vi "HEWH RLT PRAT.vi"() -> ()   [LabVIEW 2023] (continued)
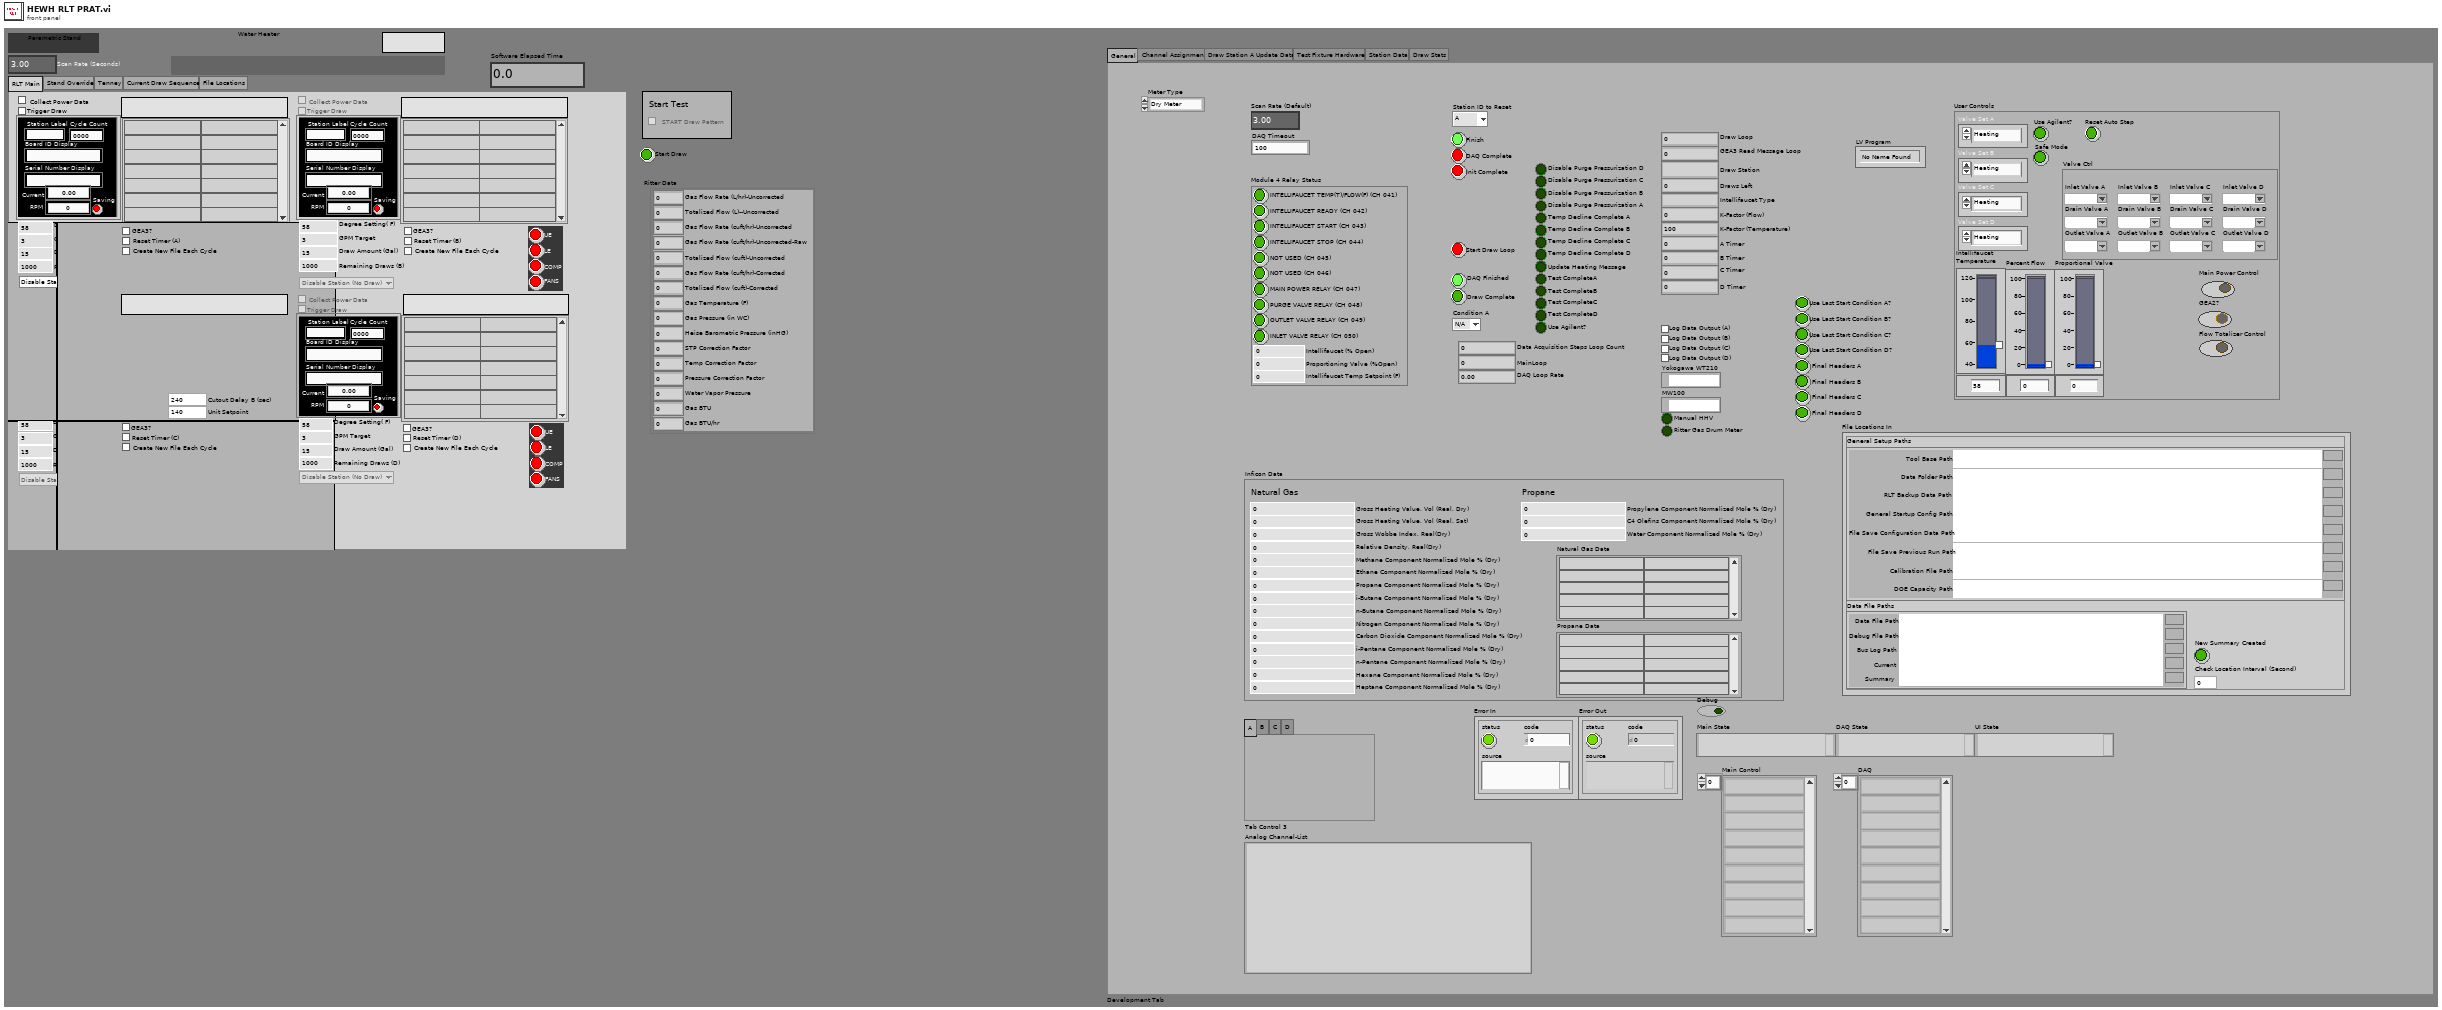
[diagram p1: front panel]
types:
  T1 = typedef "Ritter Data.ctl" = cluster{"Gas Flow Rate (L/hr)-Uncorrected":dbl, "Totalized Flow (L)--Uncorrected":dbl, "Gas Flow Rate (cuft/hr)-Uncorrected":dbl, "Totalized Flow (cuft)-Uncorrected":dbl, "Gas Temperature (F)":dbl, "Gas Pressure (in WC)":dbl, "Heise Barometric Pressure (inHG)":dbl, "STP Correction Factor":dbl, "Temp Correction Factor":dbl, "Pressure Correction Factor":dbl, "Water Vapor Pressure":dbl, "Gas Flow Rate (cuft/hr)-Corrected":dbl, "Totalized Flow (cuft)-Corrected":dbl, "Gas BTU":dbl, "Gas BTU/hr":dbl, "Gas Flow Rate (cuft/hr)-Uncorrected-Raw":dbl}
  T2 = typedef "HEWH Special Condition Check.ctl" = enum16{"N/A", "C1", "C2", "Reset/Fail", "Skip Draw Sequence"}
  T3 = typedef "File Setup.lvlib/Save File DOE File Path Control.ctl" = cluster{"General Setup Paths":cluster{"Calibration File Path":path, "DOE Capacity Path":path, "Data Folder Path":path, "RLT Backup Data Path":path, "Tool Base Path":path, "General Startup Config Path":path, "File Save Previous Run Path":path, "File Save Configuration Data Path":path}, "Data File Paths":T4, "New Summary Created":bool, "Check Location Interval (Second)":i32}
  T4 = typedef "File Setup.lvlib/Save File DOE Data Save Filepaths.ctl" = cluster{"Data File Path":path, "Debug File Path":path, "Bus Log Path":path, "Current":path, "Summary":path}
  T5 = typedef "File Setup.lvlib/Save File DISH Dishwasher Details.ctl" = cluster{"FileVersionInfo":T6, "Dishwasher Info":cluster{"Open Cup Weight (gm):":dbl, "Auto Cup Weight (gm):":dbl, "Detergent-Dish:":string, "Inlet Temperature-Dish:":string, "Cycle Mode-Dish:":string, "Unit Control-Dish:":string, "Manufacturer-Dish:":string}, "Washer Info":cluster{"Hot Water Temperature (Fahrenheit):":string, "Cold Water Temperature (Fahrenheit):":string, "Capacity (cu.ft):":dbl, "Initial Cloth Weight:":dbl, "Cloth Lot:":i32, "Model Family:":string, "Program Name:":string, "Cycle Selection:":string, "Wash Temperature:":string, "Rinse Temperature:":string, "Load Size:":string}, "File Name Output Array":string[][], "Calibration Output Array":string[][], "Appliance Common":T7, "Water Heater":cluster{"Heating Mode:":string}, "Dryer":cluster{"Heat Setting:":T8, "Washer Water Temperature (60 ± 5°F):":u16, "Water Hardness (PPM):":u16, "Dryness Setting:":T8, "Dryer Type:":string, "Exhaust:":string, "Drying Cycle:":string, "Load Type:":string, "Nominal Load Weight":string, "Dryer Initial IMC Data":T9}}
  T6 = typedef "FileVersionInformation.ctl" = cluster{"FileVersion":string, "ProductName":string, "InternalName":string, "CompanyName":string, "LegalCopyright":string, "FileDescription":string}
  T7 = typedef "DOE Appliance Common.ctl" = cluster{"Engineer:":string, "Model Number:":string, "Serial Number:":string, "Comments:":string, "Station ID:":string, "Technician:":string, "TR Number:":string, "Lab ID:":string, "Voltage:":string, "Water Pressure (PSI):":string, "Test Date:":string, "Computer Name:":string, "IP Address:":string, "Ambient RH:":string, "Frequency:":string, "Build:":string, "Filename:":string, "Test Type:":string, "Load Run #:":i32, "Ambient Temperature (F):":string, "File Path:":path, "Cycles Per Year":u32}
  T8 = typedef "Custom Pallet String.ctl" = string
  T9 = typedef "DPT IMC Data.ctl" = cluster{"Measured IMC (lbs)":dbl, "Actual Initial RMC (%)":dbl, "RMC (Desired %)":dbl, "Bone Dry Wt(lbs)":dbl, "Tolerance(%)":dbl, "Actual Final RMC (%)":dbl, "CEF (lbf/kWh)":dbl, "Minimum Weight (lbf)":dbl, "Average Weight (lbf)":dbl, "Maximum Weight (lbf)":dbl, "Measured IMC In Range?":bool, "Moisture Reduction Factor":dbl, "Field Use Factor":dbl, "Empty Dryer Cold Weigth":dbl, "Energy Standard":T10, "Weight Cloth (lbs)":dbl, "Relative Moisture Content (%)":dbl, "Relative Moisture Content - Avg (%)":dbl}
  T10 = typedef "DOE Dryer Standard.ctl" = enum16{"D2-Automatic Dryer", "D2-Timer Dryer", "D1-Automatic Dryer", "D1-Timer Dryer", "Other"}
  T11 = typedef "Custom Pallet DBL.ctl" = dbl
  T12 = typedef "UTILITY Power Analyzer.ctl" = enum16{"", "APLUS", "WT210", "WT500", "WT300", "OSI", "Debug", "WT230", "WT300_1", "WT300_2"}
  T13 = typedef "HEWH Output Information.ctl" = cluster{"Scan Rate Adjust":dbl, "Draw Count":i32, "Test Patten Setup":T14, "HEWH Specific DAQ":T21, "Test Output Data":cluster{"PreDraw Data Table":string[][], "Data Table":string[][], "MW100 TC Headers":string[]}, "Calc and Calibration":T24, "Current Draw Time":dbl, "LV Program":T25, "Station ID":T26, "Current Cond":T2, "Test Complete":bool, "ANSI Rate":T27, "Module 4 Relay Status":T28}
  T14 = typedef "HEWH Draw Pattern Setup.ctl" = cluster{"Total Gallons Schedule":dbl[], "PRAT/RLT Sequence":T15[], "Current Sequence Index":i32}
  T15 = typedef "PRAT Test.ctl" = cluster{"Sequence #":dbl, "Cycles":i32, "Mode Setting":T16, "Flow Rate (GPM)":dbl, "Temperature (F)":dbl, "Reset Timer":bool, "Use Temp Decline Method":bool, "Terminate Condition":T17, "Condition Value #1":dbl, "UE":bool, "LE":bool, "Comp":bool, "Fan":bool, "Test End Time (Sec)":dbl, "Purge Until Cutout":bool, "Start Conditions":T18, "Condition Value #2":dbl, "Remove Power":bool, "Time":dbl, "Check Special Cond.":T19, "Condition#":T2, "Draw Flags":T20, "Data Processing Delay (FHD 15sec, UEF 5 Sec)":dbl, "Test Complete":bool, "User Setpoint":dbl, "Tank Setpoint":dbl}
  T16 = typedef "File Setup.lvlib/Save File HEWH Heating Control Mode.ctl" = string
  T17 = typedef "Terminate Draw Conditions.ctl" = enum16{"C1-Terminate Draw @ Gallon Mark", "C2-Special Last Draw (HU Test)", "C3-RTD Out <=", "C4-Mean Tank Temp <=", "C5-Decrease RTD Out (Deg F)", "C6-Time (Seconds)", "C7-Until Any Heat Source", "C8-Specific Heat Source", "C9-Do Nothing", "C10-Inlet Outlet RTD Temp Delta"}
  T18 = typedef "HEWH Start Conditions.ctl" = enum16{"Heat Source Cutout", "At Time (Seconds)", "Every X (Seconds)", "T2 >= X° Below Setpoint", "Seconds From Complete", "Wait for LE & Comp Cutout", "Wait for Comp Cutout", "Wait for LE Cutout", "Wait for UE Cutout", "Start Immediately"}
  T19 = typedef "Check Special Condtions.ctl" = enum16{"SC1-Do Nothing", "SC2-Check Heat Source (On-C2/Off-C1)", "SC3-Check Skip Condition", "SC4-Check Heat Source ON/Fail", "SC5-Keep Draw Valves Open", "SC6-Skip Purge"}
  T20 = typedef "HEWH Draw Flag ENUM.ctl" = enum16{"N/A", "None(0)", "Sml(1)", "Med(2)", "SmlMed(3)", "Lrg(4)", "SmlLrg(5)", "MedLrg(6)", "SmlMedLrg(7)"}
  T21 = typedef "HEWH Specific DAQ.ctl" = cluster{"HEWH Data":T22, "Flow Valve % Open":dbl, "Power State":T23, "Power Analyzer":T12, "Flow Valve uA Output":i32, "Gallons Start (Gal)":dbl, "PI Output":dbl}
  T22 = typedef "HEWH Power Data.ctl" = cluster{"HEWH Standard":cluster{"Voltage (Volts)":dbl, "Current (Amps)":dbl, "Power (Watts)":dbl, "WattHours (Wh)":dbl, "TC Tree (AVG)":dbl, "Flow Rate (GPM)":dbl, "Gallons (Gal)":dbl, "RTD Out (Deg F)":dbl, "RTD In (Deg F)":dbl, "RTD Amb (Deg F)":dbl, "TC Down":dbl, "UE Event Lead":i32, "LE Event Lead":i32, "TC 8":dbl, "TC 9":dbl, "TC 10":dbl, "TC Tree Array (1-6)":dbl[], "TC 7":dbl, "PSI 1":dbl, "PSI 2":dbl, "PSI 3":dbl, "PSI 4":dbl}, "PRAT":cluster{"Power (Watts) A":dbl, "Power (Watts) B":dbl, "Power (Watts) C":dbl, "Power (Watts) D":dbl, "TC1":dbl, "TC2":dbl, "TC3":dbl, "TC4":dbl, "WattHours (Wh) A":dbl, "WattHours (Wh) B":dbl, "WattHours (Wh) C":dbl, "WattHours (Wh) D":dbl, "Ambient":dbl, "Extra Temp":dbl}, "Additional Power Data":cluster{"Vthd":dbl, "Frequency (Hz)":dbl, "Apparent Power (VA)":dbl, "Power Factor":dbl, "Current Crest Factor":dbl, "Voltage Crest Factor":dbl, "Integration Time (sec)":dbl}}
  T23 = typedef "HEWH Power Elements.ctl" = cluster{"UE":bool, "LE":bool, "COMP":bool, "FANS":bool}
  T24 = typedef "HEWH Calc and Calibration.ctl" = cluster{"Mean SD Var Max Min Array":string[][], "Draw Statistics (DBL)":dbl[][], "Calibration Coefficients DBL":dbl[][], "Start Gallons":dbl, "Starting Temp Decline":dbl, "K-Factor (Temperature)":dbl, "All Draw Stats":string[][], "RTD Terminate Value":dbl, "K-Factor (Flow)":dbl, "Intellifaucet Type":string, "Thermal Stabil Array":dbl[][], "Gas Thermal Stabil Complete":bool, "Therm Reset Cmpt 1":bool, "Therm Reset Cmpt 2":bool, "Last Flow Rate (Therm)":dbl, "State":enum16{"State 0", "State 1", "State 2", "State 3", "State 4", "State 5", "State 6"}, "Gas Thermal Time":dbl, "Target Rate (Thermal)":dbl, "Thermal - Final":dbl[][], "State5 Gal Water":dbl, "State 5 Gal Gas":dbl, "Intellif Open < 1":dbl, "Intellif Open < 1.7":dbl, "Intellif Open < 2.2":dbl, "Intellif Open > 2.2":dbl, "End of Draw\nComparison":bool[][], "Temperature Decline Method":cluster{"Previous Cycle Count":i32, "Previous Max Temp In":dbl, "Previous Trigger In":u8, "Start Timer":dbl, "first_iteration":dbl}}
  T25 = typedef "File Setup.lvlib/Save File DOE LabView Program.ctl" = enum16{"No Name Found", "DOE Stand", "Dishwasher Kitchen", "Portable Stand", "HEWH", "Dryer", "Dryer WILT", "HCC", "PRAT", "HEWH RLT", "Refrigeration", "Gas Water Heater"}
  T26 = typedef "Station ID Selector.ctl" = enum16{"", "A", "B", "C", "D", "Global"}
  T27 = typedef "RANGE ANSI Rate.ctl" = cluster{"Array 1":dbl[], "Array 3":dbl[], "Array 2":dbl[], "Start ANSI":bool, "ANSI Start Time":dbl, "Restart ANSI":bool, "15 Min ANSI Avg (BTU/hr)":dbl, "20 Min ANSI Avg (BTU/hr)":dbl, "25 Min ANSI Avg (BTU/hr)":dbl, "Absolute Pressure":dbl, "Gas Temperature":dbl, "Volumetric Flow Rate":dbl, "Mass Flow Rate":dbl, "Array 4":dbl[], "Array 5":dbl[], "Gas Rate":dbl, "15 Min Pres Avg (PSIA)":dbl, "20 Min Pres Avg (PSIA)":dbl, "25 Min Pres Avg (PSIA)":dbl, "15 Min Temp Avg (°F) ":dbl, "20 Min Temp Avg (°F)":dbl, "25 Min Temp Avg (°F)":dbl, "15 Min Uncorrected Avg (CFH)":dbl, "20 Min Uncorrected Avg (CFH)":dbl, "25 Min Uncorrected Avg (CFH)":dbl, "15 Min Corrected Avg (SCFH)":dbl, "20 Min Corrected Avg (SCFH)":dbl, "25 Min Corrected Avg (SCFH)":dbl, "15 Min Complete":bool, "20 Min Complete":bool, "25 Min Complete":bool, "Heating Value (BTU/ft³)":dbl, "CO CO2 15 Min":string[][], "CO CO2 20 Min":string[][], "CO CO2 25 Min":string[][], "CO CO2 Real Time":string[][]}
  T28 = typedef "HEWH Module 4 Relay Status.ctl" = cluster{"INTELLIFAUCET TEMP(T)/FLOW(F) (CH 041)":bool, "INTELLIFAUCET READY (CH 042)":bool, "INTELLIFAUCET START (CH 043)":bool, "INTELLIFAUCET STOP (CH 044)":bool, "MAIN POWER RELAY (CH 047)":bool, "NOT USED (CH 045)":bool, "NOT USED (CH 046)":bool, "PURGE VALVE RELAY (CH 048)":bool, "OUTLET VALVE RELAY (CH 049)":bool, "INLET VALVE RELAY (CH 050)":bool, "Intellifaucet (% Open)":dbl, "Proportioning Valve (%Open)":dbl, "Intellifaucet Temp Setpoint (F)":dbl}
  T29 = typedef "Custom Pallet Timer.ctl" = dbl
  T30 = enum32{"RLT Main", "Stand Override", "Tenney", "Current Draw Sequence", "File Locations"}
  T31 = typedef "Save File.lvlib/Save File Washer.ctl" = cluster{"Appliance Details":T5, "Display Data (RLT)":T32}
  T32 = typedef "Save File Appliance Display.ctl" = cluster{"Status Color":u32, "Serial Number Display":string, "Cycle Count Display":i32, "Station Label Display":string, "Current Run Start Time Display":dbl, "Board ID Display":string, "RPM Display":u32, "Current Display":dbl, "Current Path Display":path, "Saving Display":bool, "Unit Type Display":T33, "Total Time On Display":dbl, "UI Button":bool}
  T33 = typedef "Save File.lvlib/Save File Unit Type.ctl" = enum32{"", "Viper", "Hawk", "2015"}
  T34 = typedef "HEWH RLT Station Disable.ctl" = enum16{"Disable Station (No Draw)", "Enable Station"}
  T35 = enum32{"Station A", "Station B", "Station C", "Station D"}
  T36 = typedef "HEWH Tank Indicator.ctl" = cluster{"TC1":dbl, "TC2":dbl, "TC3":dbl, "TC4":dbl, "TC5":dbl, "TIN":dbl, "TOUT":dbl, "TC6":dbl, "TC6-Color":u32, "TC5-Color":u32, "TC4-Color":u32, "TC3-Color":u32, "TC2-Color":u32, "TC1-Color":u32, "RTD-Out":u32, "RTD-In":u32}
  T37 = cluster{"Time Array Output":dbl[], "Data Array Output":dbl[]}[]
  T38 = enum32{"Quick Settings", "Manual Valve Override", "Message Screen", "GEA Commands", "Gas", "Vesta", "Enviracom"}
  T39 = typedef "HEWH Valve Bank Positions.ctl" = enum16{"Heating", "Purge", "Resting", "Draw"}
  T40 = typedef "HEWH Normally Open Valve Control.ctl" = string
  T41 = typedef "HEWH Normally Closed Valve Control.ctl" = string
  T42 = typedef "GEA3 HEWH Personality.ctl" = string
  T43 = typedef "FMA1600A Gas Type.ctl" = string
  T44 = typedef "Temperature Control.ctl" = cluster{"Water Heater Temp (°F)":u16, "Differential  (°F)":dbl}
  T45 = typedef "Burner State.ctl" = enum16{"Burner OFF", "Burner ON"}
  T46 = typedef "Tenney Chamber Status.ctl" = enum16{"OFF", "ON"}
  T47 = typedef "Tenney Temperature Limits.ctl" = cluster{"Target Temperature Upper limit":dbl, "Target Temperature Lower limit":dbl, "Target Humidity Lower limit":dbl, "Target Humidity Upper limit":dbl, "Chamber Temperature Upper limit":dbl, "Chamber Temperature Lower limit":dbl, "Chamber Humidity Lower limit":dbl, "Chamber Humidity Upper limit":dbl, "Chamber Adjustment Increment (F)":dbl, "Chamber Adjustment Interval (Minutes)":dbl, "Chamber Adjustment Increment (%)":dbl, "Chamber Adjustment Interval Fast (Minutes)":dbl}
  T48 = typedef "HEWH Draw Parameters.ctl" = cluster{"Draws Left":i32, "Draws Left Array":i32[], "Remaining Draws (A)":i32, "Remaining Draws (B)":i32, "Remaining Draws (C)":i32, "Remaining Draws (D)":i32, "Index of Element (A-D)":i32[], "Station A":T15, "Station B":T15, "Station C":T15, "Station D":T15}
  T49 = typedef "HEWH GEA3 Board ID.ctl" = enum16{"Board ID - 0", "Board ID - 1", "Board ID - 2", "Board ID - 3"}
  T50 = typedef "HEWH Full Station IDs.ctl" = enum16{"Default", "1ED", "2ED", "3ED", "4ED", "6A", "6B", "6C", "6D"}
  T51 = enum32{"General", "Channel Assignment", "Draw Station A Update Data", "Test Fixture Hardware", "Station Data", "Draw Stats"}
  T52 = typedef "HEWH User Controls.ctl" = cluster{"Main Power Control":bool, "Flow Totalizer Control":bool, "Intellifaucet \nTemperature":dbl, "Percent Flow":dbl, "Safe Mode":bool, "GEA2?":bool, "Use Agilent?":bool, "Valve Set A":enum16{"Heating", "Purge", "Resting", "Draw"}, "Valve Set B":enum16{"Heating", "Purge", "Resting", "Draw"}, "Valve Set C":enum16{"Heating", "Purge", "Resting", "Draw"}, "Valve Set D":enum16{"Heating", "Purge", "Resting", "Draw"}, "Valve Ctrl":cluster{"Outlet Valve D":T40, "Drain Valve D":T41, "Inlet Valve D":T40, "Outlet Valve C":T40, "Drain Valve C":T41, "Inlet Valve C":T40, "Outlet Valve B":T40, "Drain Valve B":T41, "Inlet Valve B":T40, "Outlet Valve A":T40, "Drain Valve A":T41, "Inlet Valve A":T40}, "Proportional Valve":dbl, "Reset Auto Step":bool}
  T53 = typedef "Inficon Data.ctl" = cluster{"Gross Heating Value, Vol (Real, Dry)":dbl, "Nitrogen Component Normalized Mole % (Dry)":dbl, "Methane Component Normalized Mole % (Dry)":dbl, "Carbon Dioxide Component Normalized Mole % (Dry)":dbl, "Ethane Component Normalized Mole % (Dry)":dbl, "Propane Component Normalized Mole % (Dry)":dbl, "i-Pentane Component Normalized Mole % (Dry)":dbl, "i-Butane Component Normalized Mole % (Dry)":dbl, "n-Butane Component Normalized Mole % (Dry)":dbl, "n-Pentane Component Normalized Mole % (Dry)":dbl, "Hexane Component Normalized Mole % (Dry)":dbl, "Heptane Component Normalized Mole % (Dry)":dbl, "Gross Wobbe Index, Real(Dry)":dbl, "Relative Density, Real(Dry)":dbl, "Propylene Component Normalized Mole % (Dry)":dbl, "C4 Olefins Component Normalized Mole % (Dry)":dbl, "Water Component Normalized Mole % (Dry)":dbl, "Gross Heating Value, Vol (Real, Sat)":dbl, "Natural Gas Data":string[][], "Propane Data":string[][]}
  T54 = typedef "HEWH RLT MW100 Station Channels.ctl" = cluster{"MW100":cluster{"Station A Channels, MW100":string[][], "Station B Channels, MW100":string[][], "Station C Channels, MW100":string[][], "Station D Channels, MW100":string[][]}, "Agilent":cluster{"Station A Channels, Agilent":string[][], "Station B Channels, Agilent":string[][], "Station C Channels, Agilent":string[][], "Station D Channels, Agilent":string[][]}}
  T55 = typedef "DOE Test Fixture Hardware.ctl" = cluster{"Power ":T56, "Weight Scale":cluster{"Com Options":T57, "Select Scale":string}, "Flow Rates":cluster{"Laurel Cold IP Address":string, "Laurel Hot IP Address":string, "Hot Water Laurel VISA":refnum<visa-resource-name>, "Cold Water Laurel VISA":refnum<visa-resource-name>, "Remote Port":u16, "Laurel Communication Type":string, "Meters To Collect (Hot Cold)":string, "HOT Laurel Reference":refnum<k5>, "COLD Laurel Reference":refnum<k5>, "Modbus Hot Ref":refnum<class "Modbus Master.lvclass">}, "Analog Data":cluster{"Agilent":cluster{"Agilent 34972_1":refnum<visa-resource-name>, "Agilent 34972_2":refnum<visa-resource-name>, "Agilent 34972_3":refnum<visa-resource-name>, "Agilent 34972_4":refnum<visa-resource-name>, "Agilent 34972_5":refnum<visa-resource-name>, "Agilent 34972_6":refnum<visa-resource-name>, "Agilent Gain":dbl, "TC Type (K,J,T)":string, "Instrument IDN?":string, "TC Channels-List":string, "Analog Channels-List":string, "Agilent Cluster Array":T58[], "TC Channels-List 2":string, "Analog Channels-List 2":string}, "Yokogawa":cluster{"MW100":refnum<visa-resource-name>, "Intellifaucet":bool}, "Select Analog":string, "TC Coefficients":T59, "NI Tasks (Dryer DOE)":refnum<k21>[], "Laurel Analog":cluster{"Laurel IP (Water Temp)":string, "Laurel IP (Pressure)":string}}, "Viasala Temperature & Humidity":cluster{"IP Address 1":string, "Remote Port":u16, "IP Address 2":string, "IP Address 3":string, "Viasala Modbus":refnum<class "Modbus Master.lvclass">, "Probe Number":u16}, "Gas Meter":T60, "Barometric Pressure":cluster{"HEISE 901A":refnum<visa-resource-name>, "Use Barometer?":bool}, "Gas Analysis":cluster{"Ultramat 23 VISA":refnum<visa-resource-name>}, "Inficon Micro GC":T64, "Tenney Environmental Chamber":cluster{"Remote Port":u16, "IP Address":string, "Tenney Modbus":refnum<class "Modbus Master.lvclass">}}
  T56 = typedef "UTILITY Power Inputs Control.ctl" = cluster{"Yokogawa":cluster{"WT210":cluster{"Sample Rate (1: 0.25s)":i32, "A Range (12: 20A)":i32, "V Range (6: 600V)":i32, "Power VISA Yokogawa WT210":refnum<visa-resource-name>}, "WT500":cluster{"Power VISA Yokogawa WT500":refnum<visa-resource-name>, "V Range (8: 1000V)":i32, "I Range (7: 40A)":i32, "Update Rate (3: 500ms)":i32}, "WT310_2":cluster{"Sample Rate (1: 0.25s)":i32, "A Range (12: 20A)":i32, "V Range (6: 600V)":i32, "Power VISA Yokogawa WT310_2":refnum<visa-resource-name>}, "WT310_3":cluster{"Sample Rate (1: 0.25s)":i32, "A Range (12: 20A)":i32, "V Range (6: 600V)":i32, "Power VISA Yokogawa WT310_3":refnum<visa-resource-name>}}, "Aplus":cluster{"Aplus IP Address":string, "Remote Port":i32, "Instrument":string, "Instr Driver Revision":string}, "Power Limits":cluster{"Crest Factor":cluster{"Upper Limit":dbl, "Lower Limit":dbl}, "Harmonic Content":cluster{"Uthd":dbl}, "Voltage":cluster{"% Error":dbl}, "Stability":cluster{"<1 Watt ":cluster{"Wattage":dbl, "Slope (mW/H)":dbl}, ">1 Watt":cluster{"1%Power/Hour":dbl}}}, "Nominal Voltage":i32, "Time Limit (s)":dbl, "Power Variation Limit (%)":dbl, "Power Supply":cluster{"Chroma 61605":refnum<visa-resource-name>, "Use Chroma?":bool}}
  T57 = typedef "IND560 Configuration.ctl" = cluster{"IND560Scale VISA":refnum<visa-resource-name>, "IP Address":string, "Remote Port":u16, "Setra Scale VISA":refnum<visa-resource-name>, "GSE 350":refnum<visa-resource-name>}
  T58 = typedef "HEWH Agilent Cluster.ctl" = cluster{"Label":string, "Agilent Channel":string, "Panel ID":string, "Source":string, "Temperature":dbl}
  T59 = typedef "UTILITY TC Coefficients.ctl" = cluster{"TC Coefficients 1":dbl[], "TC Coefficients 2":dbl[], "TC Coefficients 3":dbl[], "TC Coefficients 4":dbl[], "TC Coefficients 5":dbl[], "TC Coefficients 6":dbl[], "TC Coefficients 7":dbl[]}
  T60 = typedef "FMA1600A COM Ports.ctl" = cluster{"Gas Meter 1":refnum<visa-resource-name>, "Gas Meter 2":refnum<visa-resource-name>, "Gas Meter 3":refnum<visa-resource-name>, "Gas Meter 4":refnum<visa-resource-name>, "Gas Meter 5":refnum<visa-resource-name>, "Gas Meter 6":refnum<visa-resource-name>, "Data Frame Format":T61, "Measurement Units":T62, "Ritter Gas Meter 1":refnum<visa-resource-name>}
  T61 = typedef "Data Frame.ctl" = cluster{"Absolute Pressure":bool, "Gauge/Diff. Pressure":bool, "Barometric Pressure":bool, "Temperature":bool, "Volumetric":bool, "Mass":bool, "Setpoint":bool, "Valve Drive":bool, "Totalizer":bool, "Totalizer Timer":bool, "Totalizer Average Flow":bool, "Totalizer Peak Flow":bool, "Gas Selected":bool, "Tot. Timer Format":u16}
  T62 = typedef "FMA1600A Units String.ctl" = cluster{"Software Rev":string, "Model Number":string, "Manufacturer Info":string, "Software Sub-Rev":string, "Board Rev":string, "Units of Measure Input":T63}
  T63 = typedef "Units of Measure.ctl" = cluster{"Abs. Pressure":string, "Gauge/Diff. Press.":string, "Barometric Press.":string, "Temperature":string, "Volume":string, "Mass":string, "Setpoint":string, "Valve Drive":string, "Totalizer":string, "Tot. Timer":string, "Tot. Avg. Flow":string, "Tot. Peak Flow":string}
  T64 = typedef "Inficon IP Address.ctl" = cluster{"Propane IP Address":string, "Natural Gas  IP Address":string, "Remote Port":u16, "Natural Modbus":refnum<class "Modbus Master.lvclass">, "Propane Modbus":refnum<class "Modbus Master.lvclass">}
  T65 = typedef "Data Cluster.ctl" = cluster{"Absolute Pressure":dbl, "Gauge/Diff. Pressure":dbl, "Barometric Pressure":dbl, "Temperature":dbl, "Volumetric Flow":dbl, "Mass Flow":dbl, "Setpoint":dbl, "Valve Drive":dbl, "Totalizer":dbl, "[hr]":dbl, "[min]":dbl, "[sec]":dbl, "Totalizer Average Flow":dbl, "Totalizer Peak Flow":dbl, "Gas selected":string}
  T66 = typedef "Vesta Info.ctl" = cluster{"Temp_W_Raw_U":u16, "Temp_W_Raw_L":u16, "Temperature Water (F)":dbl, "Temperature Water Compensated (F)":dbl, "Temperature Ambient (F)":dbl, "Setpoint Location (F)":dbl, "Heat Request":string, "Fault Ram":string, "PWM DCDC Value":u16, "Pilot Voltage (mV)":dbl, "Setpoint Actual (F)":dbl, "Differential Actual (F)":dbl, "Setpoint User (F)":dbl, "Differential User (F)":dbl, "Termperature FIltered -TCO (F)":dbl, "Temp_C_Raw_1 - Sensor Voltage":string, "Temp_C_Raw_2 - Sensor Voltage":string, "Chamber Sensor Temperature (F)":dbl, "LDO Base Temperature (F)":dbl, "LDO Timer (sec)":i16, "Disabled (0)":bool, "Warming (1)":bool, "Heating (2)":bool, "Cooling Data Write (3)":bool, "Cooling (4)":bool, "Data Read (5)":bool, "N/A":bool, "Temperature Trip (7)":bool, "Burner":bool}
  T67 = typedef "Tenney UI Data.ctl" = cluster{"Timer Data":T68, "Tenney Data":T69, "Viasala Data Output":T70, "Alicat Data":T71, "Inficon Data":T53, "Inficon Data LP":T53, "Ultramat 23 Data":string[][], "Ritter Data":T1, "Heise Data":dbl, "Emerson Data":T72, "Laurel Meter Data":T73, "WT300 Data":T74, "Agilent Data":T75, "GEA Data - Station A":T76, "GEA Data - Station B":T76, "GEA Data - Station C":T76, "GEA Data - Station D":T76, "MW100 Data":T79, "Vesta Data Output":T66}
  T68 = typedef "HEWH Timer.ctl" = cluster{"Station A-Timer":string[][], "Station B-Timer":string[][], "Station C-Timer":string[][], "Station D-Timer":string[][], "Timer A":dbl, "Timer B":dbl, "Timer C":dbl, "Timer D":dbl, "TimerA (String)":string, "TimerB (String)":string, "TimerC (String)":string, "TimerD (String)":string, "TimerA (H:M:S)":string, "TimerB (H:M:S)":string, "TimerC (H:M:S)":string, "TimerD (H:M:S)":string}
  T69 = typedef "Tenney Environmental Chamber Data.ctl" = cluster{"Temperature Setpoint":dbl, "Temperature Process Variable":dbl, "Humidity Setpoint":dbl, "Humidity Process Variable":dbl, "Frequency Setpoint":dbl, "Frequency Process Variable":dbl, "Chamber Status (ON/OFF)":string}
  T70 = typedef "Viasala Indigo 520 Data.ctl" = cluster{"Temperature Probe 1":dbl, "Humidity Probe 1":dbl, "Temperature Probe 2":dbl, "Humidity Probe 2":dbl}
  T71 = typedef "Alicat Gas Meter Data.ctl" = cluster{"Data Cluster":T65, "Units of Measure Input":T63, "Header Array":string[]}
  T72 = typedef "Emerson 5700 Data.ctl" = cluster{"Mass Flow Rate (Scaled Integer)":u16, "Density (Scaled Integer)":u16, "Temperature (Scaled Integer)":u16, "Volume Flow Rate (Scaled Integer)":u16, "Totalizer 1 (Scaled Integer)":u16, "Totalizer 2 (Scaled Integer)":u16, "Transmitter Software Rev":u16, "Flow Direction":string, "Mass Flow Units":string, "Density Units":string, "Temperature Units":string, "Volume Flow Units":string, "Pressure Units":string, "Mass Total Units":string, "Volume Total Units":string, "Inventory 1 (Scaled Integer)":u16, "Inventory 2 (Scaled Integer)":u16, "Mass Flow Rate":dbl, "Density":dbl, "Temperature":dbl, "Volume Flow Rate":dbl, "Pressure (Scaled Integer)":u16, "Current Value Totalizer 1 (Pounds per draw)":dbl, "Current Value Totalizer 2 (Gallons per draw)":dbl, "Current Value Inventory 1 (Pounds Total)":dbl, "Current Value Inventory 2 (Gallons Total)":dbl, "Drive Gain":dbl, "Raw Tube Frequency (Hz)":dbl, "Dynamic Viscosity (Centipoise)":dbl, "Kinematic Viscosity (Centistokes)":dbl, "Hot Gallons (Calculated Gallons)":dbl, "Hot Flow Rate (Calculated GPM)":dbl, "Hot Gallons Inventory (Gallons)":dbl, "Hot Flow Rate (Laurel)":dbl, "Hot Gallons (Laurel)":dbl}
  T73 = typedef "Laurel Meter Data.ctl" = cluster{"Flow Rate (GPM)":dbl, "Totalized Flow (Gallons)":dbl}
  T74 = typedef "UTILITY Power Data.ctl" = cluster{"Current (A):Element 1":dbl, "Current (A):Element 2":dbl, "Power (W):Sigma":dbl, "Watt Hours (Wh):Sigma":dbl, "Voltage (V):Element 2":dbl, "Voltage (V):Element 1":dbl, "Current Crest Factor:Element 1":dbl, "Current Crest Factor:Element 2":dbl, "Voltage Harmonic (%):Element 1":dbl, "Voltage Harmonic (%):Element 2":dbl, "Voltage Crest Factor:Element 1":dbl, "Voltage Crest Factor:Element 2":dbl, "Time:Element 1":dbl, "Frequency (Hz):Element 1":dbl, "Apparent Power (VA):Element 1":dbl, "Apparent Power (VA):Element 2":dbl, "Power Factor:Element 1":dbl, "Power Factor:Element 2":dbl, "Max Watt Hours":dbl, "Voltage (V):Element 2 Avg":dbl, "Voltage (V):Element 1 Avg":dbl}
  T75 = typedef "HEWH Agilent Data.ctl" = cluster{"Location 11 (Channel 111)":dbl, "Location 12 (Channel 112)":dbl, "Location 13 (Channel 113)":dbl, "Location 14 (Channel 114)":dbl, "Location 15 (Channel 115)":dbl, "Location 16 (Channel 116)":dbl, "Location 17 (Channel 109)":dbl, "Location 18 (Channel 110)":dbl, "Location 19 (Channel 201)":dbl, "Location 20 (Channel 202)":dbl, "Location 21 (Channel 203)":dbl, "Location 22 (Channel 204)":dbl, "Location 23 (Channel 205)":dbl, "Location 24 (Channel 206)":dbl, "Location 25 (Channel 207)":dbl, "Location 26 (Channel 208)":dbl, "Location 27 (Channel 209)":dbl, "Location 28 (Channel 210)":dbl, "Location 29 (Channel 211)":dbl, "Location 30 (Channel 212)":dbl, "Location 31 (Channel 213)":dbl, "Location 32 (Channel 214)":dbl, "Location 33 (Channel 215)":dbl, "Location 34 (Channel 216)":dbl, "Location 35 (Channel 107)":dbl, "Location 36 (Channel 108)":dbl, "Location 37 (Channel 301)":dbl, "Location 38 (Channel 302)":dbl, "Location 39 (Channel 303)":dbl, "Location 40 (Channel 304)":dbl, "Location 41 (Channel 305)":dbl, "Location 42 (Channel 306)":dbl, "Location 43 (Channel 307)":dbl, "Location 44 (Channel 308)":dbl, "Location 45 (Channel 309)":dbl, "Location 46 (Channel 310)":dbl, "Location 47 (Channel 311)":dbl, "Location 48 (Channel 312)":dbl, "Location 49 (Channel 313)":dbl, "Location 50 (Channel 314)":dbl, "Location 51 (Channel 315)":dbl, "Location 52 (Channel 316)":dbl, "Location 53 (Channel 105)":dbl, "Location 54 (Channel 106)":dbl}
  T76 = typedef "HEWH GEA3 Data.ctl" = cluster{"ERD Data Input":T77, "ERD Data":string[][]}
  T77 = typedef "GEA3 HEWH ERD Data.ctl" = cluster{"Mixing Valve":T78, "Standard ERDs":cluster{"User UI Mode (0X4020)":string, "User Setpoint (0x4024)":u16, "Compressor (0x4068)":bool, "Lower Element (0x4068)":bool, "Upper Element (0x4068)":bool, "Fan (0x4068)":bool, "T1 Temp Lower Tank (°F) - (0x405F)":dbl, "T2 Temp Upper Tank (°F) - (0x4060)":dbl, "Line Voltage (0x4066)":u16, "MeasuredCurrent (0x4065)":dbl, "Tank Setpoint (°F) - (0x4026)":u16, "Depletion - (0x40CB)":u16, "Personality - (0x0035)":u16}, "Heat Pump":cluster{"EEV Position - (0X4067)":u16, "T3A TEMP EVAP IN (°F) - (0x4061)":dbl, "T3B TEMP EVAP OUT (°F) -(0x4062)":dbl, "T4 TEMP COMP DISCHARGE (°F) - (0x4063)":dbl, "T5 TEMP AMBIENT (°F)- (0x4064)":dbl, "Condensate Sensor - (0x40BC)":u16, "Fan (RPM) - (0xF073)":u16, "PWM (%) - (0xF056)":u16, "Compressor Speed (RPM) - (0xF093)":u16, "Compressor Target (RPM) - (0xF081)":u16, "Compressor Power (W) - (0xF092)":u16, "CPU Temperature (°F) - (0x40BA)":dbl, "Board Temperature (°F) - (0x40BB)":dbl}, "Inverter":cluster{"Inverter IGBT Temp (°C) - (0xF280)":dbl, "Inverter Chip Temp (°C) - (0xF284)":dbl}}
  T78 = typedef "GEA3 HEWH Mixing Valve.ctl" = cluster{"T7 Temp (°F) - (0x40B9)":dbl, "MixValveAbsoluteStepPosition - (0x400B)":i16, "Flow State - (0X4069)":u8, "T6 Temp (°F) - (0x406E)":dbl}
  T79 = typedef "HEWH MW100 Data Cluster.ctl" = cluster{"TC1-Channel 021":dbl, "TC2-Channel 022":dbl, "TC3-Channel 023":dbl, "TC4-Channel 024":dbl, "TC5-Channel 025":dbl, "TC6-Channel 026":dbl, "TC7-Channel 017":dbl, "TC8-Channel 028":dbl, "TC9-Channel 029":dbl, "TC10-Channel 030":dbl, "TC Tree Average":dbl, "TC DWN- Channel 027":dbl, "RTDin-Channel 031":dbl, "RTDout-Channel 032":dbl, "RTDamb-Channel 033":dbl, "PSI1-Channel 011":dbl, "PSI2-Channel 012":dbl, "PSI3-Channel 013":dbl, "PSI4-Channel 014":dbl, "UE State-Channel 015":dbl, "LE State-Channel 016":dbl, "Module 4 Relay Status Output":T28}
  T80 = typedef "UTILITY Notifier.ctl" = enum16{"Set", "Read", "Release Ref"}
  T81 = typedef "DRAW WATER Station Selector.ctl" = cluster{"Start Draw":bool, "Station ID":T26, "Station Draw Info":T15, "Send Condition":T2, "Disable Purge Pressurization":bool}
  T82 = typedef "Save File RLT Station Type.ctl" = enum16{"Single Station", "Four Stations"}
  T83 = typedef "Semaphore RefNum" = refnum<k1>
  T84 = typedef "usereventprio.ctl" = enum32{"high priority", "normal priority"}
  T85 = typedef "INTELLIFAUCT Temp Flow.ctl" = enum8{"TEMP", "FLOW", "Prop Valve"}
  T86 = typedef "INTELLIFAUCET Set Mode.ctl" = enum16{"Adjust Temp", "Adjust Flow", "Start Flow", "Stop Flow", "Hold Start", "Hold Stop", "Release Start", "Release Stop", "Temp/Flow Relay", "Adjust Prop Valve"}
  T87 = enum8{"Enabled", "Disabled", "Disabled and Grayed Out"}
  T88 = cluster{"Test Fixture Hardware":T55, "Save Data":string[][], "A Data Array":string[][], "B Data Array":string[][], "C Data Array":string[][], "D Data Array":string[][], "RLT Station Channels":T54, "Core HEWH Data Input A":T13, "Core HEWH Data Input B":T13, "Core HEWH Data Input C":T13, "Core HEWH Data Input D":T13, "File Locations A":T3, "File Locations B":T3, "File Locations C":T3, "File Locations D":T3, "Plot Array A":dbl[][], "Plot Array B":dbl[][], "Plot Array C":dbl[][], "Plot Array D":dbl[][]}
  T89 = typedef "DOE Main Control.ctl" = cluster{"Test Fixture Hardware":T55, "GEA2":T90, "DOE Capacity Measurments":T91, "Initialize.Washer In":T31}
  T90 = typedef "GEA2.ctl" = cluster{"Address":u8, "Source":u8, "Viper/Hawk":u8}
  T91 = typedef "DOE Capacity Measurments.ctl" = cluster{"Weight 1":dbl, "Model Number 1":string, "Temp 1":dbl, "Serial Number 1":string, "Lab Number 1":string, "Lab Number 2":string, "Serial Number 2":string, "Temp 2":dbl, "Model Number 2":string, "Weight 2":dbl, "Lab Number 3":string, "Serial Number 3":string, "Temp 3":dbl, "Model Number 3":string, "Weight 3":dbl, "Lab Number 4":string, "Serial Number 4":string, "Temp 4":dbl, "Model Number 4":string, "Weight 4":dbl, "Capacity Measurment Output String":string[][]}
  T92 = typedef "File Setup.lvlib/Save File DOE Configuration State.ctl" = enum16{"Open Front Panel", "Load Config"}
  T93 = typedef "Flow Meter Selector.ctl" = enum16{"Hot and Cold", "Hot", "Cold", "None"}
  T94 = enum32{"invalid app kind", "Development System", "Run Time System", "Student Edition", "Embedded LabVIEW", "Evaluation", "Custom"}
  T95 = cluster{"Current VI Reference":refnum<vi>, "Close Panel on Exit?":bool}
  T96 = enum32{"Invalid", "Standard", "Closed", "Hidden", "Minimized", "Maximized"}
  T97 = cluster{"Core":cluster{"Current VI Reference":refnum<vi>, "Close Panel on Exit?":bool}, "DrawsLeft":i32[], "Error Log":errorcluster[], "RLT Station Channels":T54, "Station A Display":T31, "Station B Display":T31, "Station C Display":T31, "Station D Display":T31, "Draw Parameters Seq":T48, "Current Cond A":T2, "Current Cond B":T2, "Current Cond C":T2, "Current Cond D":T2, "Power Analyzer":T12}
  T98 = typedef "whitespace.ctl" = u16
  T99 = typedef "HEWH RLT Stations.ctl" = cluster{"MW100 Labels_Channels":T100[], "Agilent Labels_Channels":T100[]}
  T100 = typedef "HEWH Label Channel.ctl" = cluster{"Label":string, "Channel":string}
  T101 = typedef "Tenney Message Queue.lvlib/All Message Queues.ctl" = cluster{"UI":refnum<queue>, "Tenney Chamber":refnum<queue>, "Viasala Humidity":refnum<queue>, "Alicat_GasMeter":refnum<queue>, "Inficon_NG":refnum<queue>, "Ultramat 23":refnum<queue>, "Ritter GasMeter":refnum<queue>, "Heise Barometer":refnum<queue>, "Inficon_LP":refnum<queue>, "Emerson":refnum<queue>, "Laurel":refnum<queue>, "WT300":refnum<queue>, "34972A":refnum<queue>, "GEA3-Station A":refnum<queue>, "GEA3-Station B":refnum<queue>, "GEA3-Station C":refnum<queue>, "GEA3-Station D":refnum<queue>, "MW100":refnum<queue>, "VestaCom":refnum<queue>, "EnviraCom":refnum<queue>, "Timer":refnum<queue>}
  T102 = typedef "HEWH Alarms.ctl" = cluster{"EEV Over A":bool, "EEV Over B":bool, "EEV Over C":bool, "EEV Over D":bool, "T-Out Over A":bool, "T-Out Over B":bool, "T-Out Over C":bool, "T-Out Over D":bool}
  T103 = cluster{"Core":cluster{"Current VI Reference":refnum<vi>, "Close Panel on Exit?":bool}, "User Controls":T52, "Test Fixture Hardware Draw Loop":T55, "Alarms":T102, "LV Program":T25, "Cal Build Array":dbl[][], "MIX VALVE STEP OFFSET":i16, "Core HEWH Data Input A":T13}
diagram:
  # "Complete"
  # "Complete"
  # "Complete"
  # "Complete"
  # "Complete"
  # "Complete"
  # "Complete"
  # "Complete"
  # "Complete. Check channels"
  # "Complete"
  # "Complete"
  # "Complete"
  # "Complete"
  # "Complete"
  # "Gradually start moving all \nDAQ components to isolated VIs. Just a lot of work. \n\nThis will improve reliability and readability"
  n1 = disable-structure shown="Disabled" {
    disable-tunnel: [w247 _] -> w103
    disable-tunnel: [w245 _] -> w102
    disable-tunnel: "Error In" -> [w244 _]
    disable-tunnel: [w241 _] -> w100
    disable-tunnel: [w233 _] -> w99
    disable-tunnel: [w217 _] -> w98
    disable-tunnel: [w216 _] -> w97
    disable-tunnel: [w211 _] -> w96
    disable-tunnel: [w200 _] -> w95
    disable-tunnel: [w187 _] -> w94
    disable-tunnel: [w186 _] -> w93
    disable-tunnel: [w185 _] -> w92
    disable-tunnel: [w184 _] -> w91
    disable-tunnel: [w183 _] -> w90
    disable-tunnel: [w170 _] -> w89
    disable-tunnel: [w169 _] -> w88
    disable-tunnel: [w168 _] -> w87
    disable-tunnel: [w167 _] -> w86
    disable-tunnel: [w166 _] -> w85
    disable-tunnel: [w165 _] -> w84
    disable-tunnel: [w131 _] -> w83
    disable-tunnel: [w130 _] -> w82
    disable-tunnel: [w109 _] -> w80
    disable-tunnel: [w108 _] -> w79
    disable-tunnel: [w107 _] -> w78
    disable-tunnel: [w106 _] -> w77
    disable-tunnel: [w104 _] -> w57
    frame Disabled {
      w201 = FALSE  # Increment Cycle
      w215 = FALSE  # Update  Sequence
      w225 = UTILITY_Notifier."Set" ("Status")
      w224 = T23 {"UE"=FALSE, "LE"=FALSE, "COMP"=FALSE, "FANS"=FALSE} ("Power Elements")
      w235 = FALSE  # Update  Cal and Calib DAQ
      w236 = FALSE  # Reset Cycle Count DAQ
      # "I dont have GEA3 working with multiple instances. This makes\nsure only Station A instance populates"
      n2 = flat-sequence {
        tunnel: ["Macro: Initialize"] -> w247
        tunnel: w244 -> [w280]
        tunnel: [w280] -> w231
        frame #0 {
          w276 = T40 "ON" ("Inlet Valve A")
          w277 = T40 "ON" ("Outlet Valve A")
          w278 = T41 "OFF" ("Inlet Valve A")
          w275 = FALSE ("Init Complete")
          w279 = FALSE ("Draw Complete")
          w281 = HEWH_RLT_Station_Disable."Disable Station (No Draw)" ("Disable Station 1")
          n3 = local write "Inlet Valve A"(w276) -> ()
          n4 = local write "Inlet Valve B"(w276) -> ()
          n5 = local write "Inlet Valve C"(w276) -> ()
          n6 = local write "Inlet Valve D"(w276) -> ()
          n7 = local write "Drain Valve B"(w278) -> ()
          n8 = local write "Drain Valve C"(w278) -> ()
          n9 = local write "Drain Valve A"(w278) -> ()
          n10 = local write "Drain Valve D"(w278) -> ()
          n11 = local write "Outlet Valve A"(w277) -> ()
          n12 = local write "Outlet Valve B"(w277) -> ()
          n13 = local write "Outlet Valve C"(w277) -> ()
          n14 = local write "Outlet Valve D"(w277) -> ()
          n15 = local write "DAQ Finished"(w279) -> ()
          n16 = local write "Draw Complete"(w279) -> ()
          n17 = local write "Shutdown"("" ("Shutdown")) -> ()
          n18 = local write "Disable Station 1"(w281) -> ()
          n19 = local write "Disable Station 2"(w281) -> ()
          n20 = local write "Disable Station 3"(w281) -> ()
          n21 = local write "Disable Station 4"(w281) -> ()
          n22 = local write "DAQ Complete"(w275) -> ()
          n23 = local write "Use Agilent?"(w275) -> ()
          n24 = local write "Init Complete"(w275) -> ()
          n25 = local write "Finish"(w275) -> ()
          n26 = local write "Start Draw Loop"(w275) -> ()
          n27 = local write "Start/Pause test"(w275) -> ()
        }
      }
      n28 = call "HEWH Power Notifier.vi"("Status"=w225, "error in (no error)"=w231, "Set Status"=w224, "name (unnamed)"="PowerA") -> ("error out"=w230:errorcluster)  [unwired: 6 in, 1 out]
      n29 = call "HEWH Power Notifier.vi"("Status"=w225, "error in (no error)"=w230, "Set Status"=w224, "name (unnamed)"="PowerB") -> ("error out"=w228:errorcluster)  [unwired: 6 in, 1 out]
      n30 = call "HEWH Power Notifier.vi"("Status"=w225, "error in (no error)"=w228, "Set Status"=w224, "name (unnamed)"="PowerC") -> ("error out"=w227:errorcluster)  [unwired: 6 in, 1 out]
      n31 = call "HEWH Power Notifier.vi"("Status"=w225, "error in (no error)"=w227, "Set Status"=w224, "name (unnamed)"="PowerD") -> ("error out"=w190:errorcluster)  [unwired: 6 in, 1 out]
      n32 = Current VI's Path() -> (path=w193:path)
      n33 = call "UTILITY This VIs Path.vi"("path"=w193, "error in (no error)"=w190) -> ("Folder Path"=w188:path, "FileVersionInfo Out"=w194:T6, "error out"=w189:errorcluster)  [unwired: 7 in, 4 out]
      n34 = Unbundle By Name(w194) -> ("FileVersion"=→"File  Version":string)
      n35 = call "HEWH Read Settings.vi"("Tool Base Path"=w188, "Error In"=w189) -> ("Intellifaucet Open Less 1 GPM"=→"Intellifaucet Open Less 1 GPM":dbl, "Ritter Gas Drum Meter"=→"Ritter Gas Drum Meter":bool, "Intellifaucet Open Less 1_7 GPM"=→"Intellifaucet Open Less 1_7 GPM":dbl, "Manual HHV"=→"Manual HHV":bool, "Intellifaucet Open Less  2.2 GPM"=→"Intellifaucet Open Less  2.2 GPM":dbl, "Intellifaucet Type"=→"Intellifaucet Type":string, "Intellifaucet Open Greater 2.2 GPM"=→"Intellifaucet Open Greater 2.2 GPM":dbl, "K-Factor (Flow)"=→"K-Factor (Flow)":dbl, "K-Factor (Temperature)"=→"K-Factor (Temperature)":dbl, "Power Analyzer"=→"Power Analyzer":T12, "Station"=→"Station":string, "LV Program"=w197:T25, "Error Out"=w198:errorcluster)  [unwired: 5 in]
      "LV Program" <- w197
      n36 = case shown="Default" w197 {
        tunnel: [Save_File_RLT_Station_Type."Single Station" ("RLT Station Type") Save_File_RLT_Station_Type."Four Stations" ("RLT Station Type")] -> w187
        frame Default {
          w271 = FALSE ("New File Per CycA")
          n37 = local write "New File Per CycB"(w271) -> ()
          n38 = local write "New File Per CycA"(w271) -> ()
          n39 = local write "New File Per CycC"(w271) -> ()
          n40 = local write "New File Per CycD"(w271) -> ()
        }
        frame "PRAT", "HEWH RLT" {
          w273 = TRUE ("New File Per CycA")
          n41 = local write "New File Per CycB"(w273) -> ()
          n42 = local write "New File Per CycA"(w273) -> ()
          n43 = local write "New File Per CycC"(w273) -> ()
          n44 = local write "New File Per CycD"(w273) -> ()
        }
      }
      n45 = call <vilib>:"Obtain Semaphore Reference.vi"("error in (no error)"=w198, "name (unnamed)"="MW100") -> ("error out"=w222:errorcluster, "semaphore"=w211:T83)  [unwired: 3 in, 1 out]
      n46 = Create User Event(user event datatype=w236, error in=w222) -> (user event=w170:refnum<user-event>, error out=w234:errorcluster)
      n47 = Create User Event(user event datatype=w235, error in=w234) -> (user event=w233:refnum<user-event>, error out=w214:errorcluster)
      n48 = Create User Event(user event datatype=w215, error in=w214) -> (user event=w169:refnum<user-event>, error out=w147:errorcluster)
      n49 = Create User Event(user event datatype=w201, error in=w147) -> (user event=w200:refnum<user-event>, error out=w196:errorcluster)
      n50 = register-events(w170, w200) -> (reference out=w216:refnum<event-registration>)  [unwired: 2 in, 1 out]
      n51 = Obtain Queue(name (unnamed)="Start Draw", element data type=T81 {"Start Draw"=FALSE, "Station ID"=enum."A", "Station Draw Info"={"Sequence #"=0.0, "Cycles"=0, "Mode Setting"="", "Flow Rate (GPM)"=0.0, "Temperature (F)"=0.0, "Reset Timer"=FALSE, "Use Temp Decline Method"=FALSE, "Terminate Condition"=enum."C1-Terminate Draw @ Gallon Mark", "Condition Value #1"=0.0, "UE"=FALSE, "LE"=FALSE, "Comp"=FALSE, "Fan"=FALSE, "Test End Time (Sec)"=0.0, "Purge Until Cutout"=FALSE, "Start Conditions"=enum."Heat Source Cutout", "Condition Value #2"=0.0, "Remove Power"=FALSE, "Time"=0.0, "Check Special Cond."=enum."SC2-Check Heat Source (On-C2/Off-C1)", "Condition#"=enum."C1", "Draw Flags"=enum."N/A", "Data Processing Delay (FHD 15sec, UEF 5 Sec)"=0.0, "Test Complete"=FALSE, "User Setpoint"=0.0, "Tank Setpoint"=0.0}, "Send Condition"=enum."N/A", "Disable Purge Pressurization"=FALSE}, error in (no error)=w196) -> (queue out=w241:refnum<queue>, error out=w149:errorcluster)  [unwired: 2 in, 1 out]
      n52 = call "UTILITY String Notifier.vi"("Status"=UTILITY_Notifier."Set", "error in (no error)"=w149, "Set Status"="", "name (unnamed)"="TimerA") -> ("error out"=w152:errorcluster)  [unwired: 6 in, 1 out]
      n53 = register-events(w233, w169) -> (reference out=w217:refnum<event-registration>)  [unwired: 2 in, 1 out]
      n54 = case shown="Default" w197 {
        tunnel: ["Data: Initialize\nUpdate File Locations\nLoad Configuration\nInitialize Equipment\nInit Hot Laurel\nUI Initialize\nData: Get MW100 (Station A)\nUI Initialize 2\nData: Get MW100 (Station A)\nUI Initialize 3\nDAQ Loop Complete" "Data: Initialize\nUpdate File Locations\nLoad Configuration\nInitialize Equipment\nDAQ Loop Complete"] -> w246
        frame Default {
        }
        frame "PRAT", "HEWH RLT" {
        }
      }
      n55 = call "UTILITY String Notifier.vi"("Status"=UTILITY_Notifier."Set", "error in (no error)"=w152, "Set Status"="", "name (unnamed)"="TimerB") -> ("error out"=w151:errorcluster)  [unwired: 6 in, 1 out]
      n56 = call "UTILITY String Notifier.vi"("Status"=UTILITY_Notifier."Set", "error in (no error)"=w151, "Set Status"="", "name (unnamed)"="TimerC") -> ("error out"=w150:errorcluster)  [unwired: 6 in, 1 out]
      n57 = call <vilib>:"Add State(s) to Queue__jki_lib_state_machine.vi"("State(s) in (\"\")"=w246) -> ("States Out"=w245:string)  [unwired: 14 in]
      n58 = call "UTILITY String Notifier.vi"("Status"=UTILITY_Notifier."Set", "error in (no error)"=w150, "Set Status"="", "name (unnamed)"="TimerD") -> ("error out"=w148:errorcluster)  [unwired: 6 in, 1 out]
      n59 = call "UTILITY String Notifier.vi"("Status"=UTILITY_Notifier."Set", "error in (no error)"=w148, "Set Status"="", "name (unnamed)"="Message") -> ("error out"=w218:errorcluster)  [unwired: 6 in, 1 out]
      n60 = call "UTILITY Boolean Notifier.vi"("Status"=UTILITY_Notifier."Set", "error in (no error)"=w218, "Set Status"=FALSE, "name (unnamed)"="Stop Custom Draw") -> ("error out"=w207:errorcluster)  [unwired: 6 in, 1 out]
      n61 = call "HEWH Draw Flag.vi"("Station ID"=Station_ID_Selector."Global", "Status"=UTILITY_Notifier."Set", "Error In"=w207) -> ("Error Out"=w206:errorcluster)  [unwired: 8 in, 4 out]
      n62 = call "HEWH Cut Out Flag.vi"("Error In"=w206) -> ("Error Out"=w202:errorcluster)  [unwired: 10 in]
      n63 = call "UTILITY Boolean Notifier.vi"("Status"=UTILITY_Notifier."Set", "error in (no error)"=w202, "Set Status"=FALSE, "name (unnamed)"="Use Last Start Condition") -> ("error out"=w174:errorcluster)  [unwired: 6 in, 1 out]
      n64 = call "HEWH GEA Notifier.vi"("Status"=UTILITY_Notifier."Set", "error in (no error)"=w174, "name (unnamed)"="GEA_A") -> ("error out"=w173:errorcluster)  [unwired: 7 in, 1 out]
